vi "OBJ_recolor_statuses.vi"(6 "Recolor? (T)":bool=TRUE, 8 "error_in":errorcluster, 11 "OBJ_all_info":T1) -> (0 "error_out":errorcluster)   [LabVIEW 2019]
uses:
  FGV/OBJ_records_display/OBJ_all_info.ctl
  OBJ_header_data_display.ctl
  OBJ_measurement_status.ctl
  FGV/OBJ_records_display/OBJ_references.ctl
panel:
  # "GEAR INFO SUMMARY"
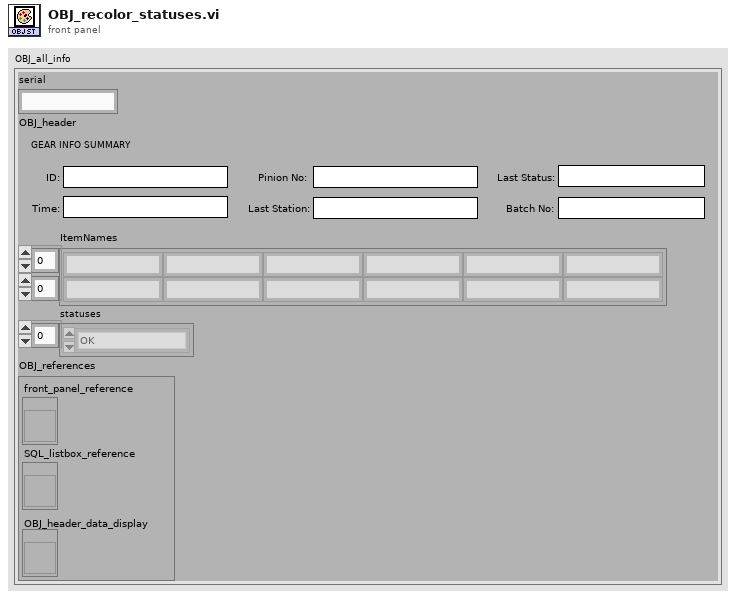
[diagram p1: front panel]
types:
  T1 = typedef "OBJ_all_info.ctl" = cluster{"serial":string, "OBJ_header":T2, "ItemNames":string[][], "statuses":T3[], "OBJ_references":T4}
  T2 = typedef "OBJ_header_data_display.ctl" = cluster{"ID":string, "creation_time":string, "last_station":string, "last_status":string, "pinion_serial":string, "batch_code":string}
  T3 = typedef "OBJ_measurement_status.ctl" = enum16{"OK", "NOK"}
  T4 = typedef "OBJ_references.ctl" = cluster{"front_panel_reference":refnum<vi>, "SQL_listbox_reference":refnum<vi>, "OBJ_header_data_display":refnum<vi>}
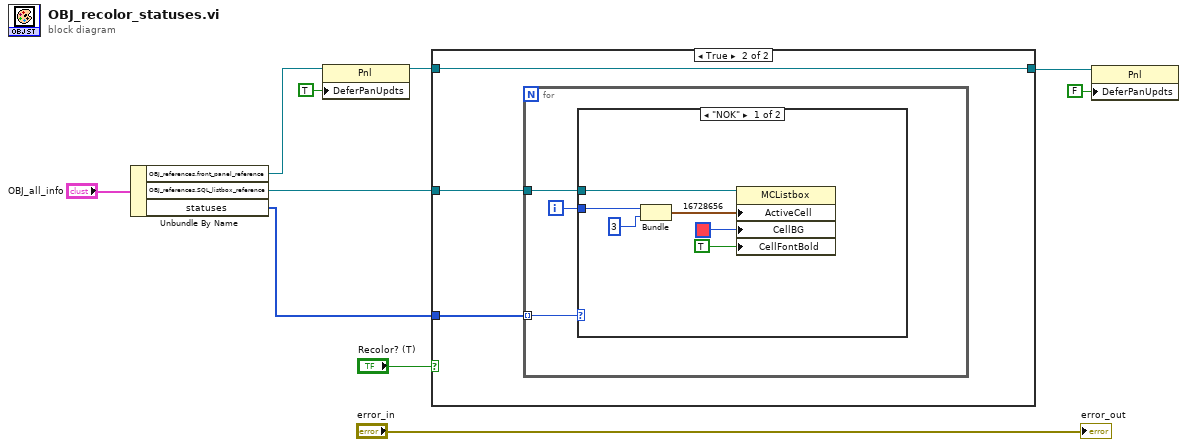
[diagram p0: block diagram]
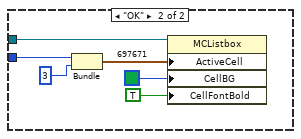
[diagram p3: hidden frame]
diagram:
  n1 = Unbundle By Name("OBJ_all_info") -> ("OBJ_references.front_panel_reference"=w7:refnum<vi>, "OBJ_references.SQL_listbox_reference"=w2:refnum<vi>, "statuses"=w1:T3[])
  n2 = property class="Pnl"(reference=w7, "DeferPanUpdts"=TRUE ("Defer Panel Updates")) -> (reference out=w5:refnum<vi>)  [unwired: 1 in, 1 out]
  n3 = case shown="True" "Recolor? (T)" {
    tunnel: w1 -> [_ w13]
    tunnel: w2 -> [_ w14]
    tunnel: w5 -> [w11 w12]
    tunnel: [w11 w12] -> w3
    frame False {
    }
    frame True {
      n4 = for {
        tunnel: w14 -> [w17]
        tunnel: w13 -> [w16] mode=indexing
        i -> [w15]
        n5 = case shown="\"NOK\"" w16 {
          tunnel: w17 -> [w21 w28]
          tunnel: w15 -> [w20 w27]
          frame "NOK" {
            n6 = Bundle(w20, 3) -> (w22:cluster{i32, i32})  [unwired: 1 in]
            n7 = property on="Property Node" class="MCListbox"(reference=w21, "ActiveCell"=w22, "CellBG"=u32 16728656, "CellFontBold"=TRUE ("Active Cell:Cell Font:Bold")) -> ()  [unwired: 1 in, 2 out]
          }
          frame "OK" {
            n8 = Bundle(w27, 3) -> (w25:cluster{i32, i32})  [unwired: 1 in]
            n9 = property on="Property Node" class="MCListbox"(reference=w28, "ActiveCell"=w25, "CellBG"=u32 697671, "CellFontBold"=TRUE ("Active Cell:Cell Font:Bold")) -> ()  [unwired: 1 in, 2 out]
          }
        }
      }
    }
  }
  n10 = property class="Pnl"(reference=w3, "DeferPanUpdts"=FALSE ("Defer Panel Updates")) -> ()  [unwired: 1 in, 2 out]
  "error_out" <- "error_in"
